vi "打开或关闭文件.vi"   [LabVIEW 2018]
types:
  T1 = enum16{"open", "replace", "create", "open or create", "replace or create", "replace or create with confirmation"}
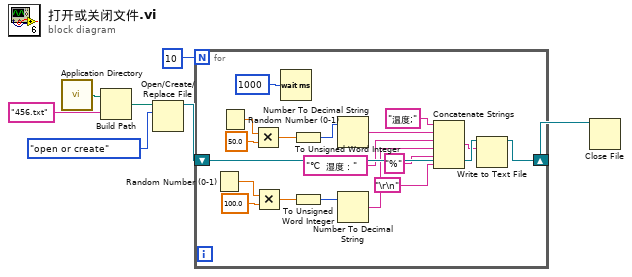
[diagram p0: block diagram]
diagram:
  n1 = call <vilib>:"Application Directory.vi"() -> ("Application Directory"=w7:path)
  n2 = Build Path(base path=w7, name or relative path="456.txt" ("名称或相对路径")) -> (appended path=w5:path)
  n3 = Open/Create/Replace File(file path (use dialog)=w5, operation (0:open)=T1."open or create" ("操作(0:open)")) -> (refnum out=w3:refnum<file>)  [unwired: 4 in, 2 out]
  n4 = for {
    N: 10 -> [_]
    shift-right: [w8] -> w1
    shift-left: w3 -> [w25]
    n5 = Random Number (0-1)() -> (number: 0 to 1=w22:dbl)
    n6 = Random Number (0-1)() -> (number: 0 to 1=w23:dbl)
    n7 = Multiply(x=w23, y=50.0) -> (x*y=w18:dbl)
    n8 = Multiply(x=w22, y=100.0) -> (x*y=w19:dbl)
    n9 = Wait (ms)(milliseconds to wait=u32 1000 ("等待时间（毫秒）")) -> ()  [unwired: 1 out]
    n10 = To Unsigned Word Integer(number=w18) -> (unsigned 16bit integer=w17:u16)
    n11 = To Unsigned Word Integer(number=w19) -> (unsigned 16bit integer=w16:u16)
    n12 = Number To Decimal String(number=w17) -> (decimal integer string=w13:string)  [unwired: 1 in]
    n13 = Number To Decimal String(number=w16) -> (decimal integer string=w12:string)  [unwired: 1 in]
    n14 = Concatenate Strings("温度;" ("字符串"), w13, "℃  湿度：" ("字符串"), w12, "%" ("字符串"), "\r\n") -> (w11:string)
    n15 = Write to Text File(file (use dialog)=w25, text=w11) -> (refnum out=w8:refnum<file>)  [unwired: 2 in, 2 out]
  }
  n16 = Close File(refnum=w1) -> ()  [unwired: 1 in, 2 out]
